vi "kloehn_error.vi"(3 "kloehn session in":T1={"VISA resource out"="COM12", "error out"={"status"=FALSE, "code"=0, "source"=""}}) -> (0 "error?":bool, 1 "kloehn session out":T1={"VISA resource out"="COM12", "error out"={"status"=FALSE, "code"=0, "source"=""}})   [LabVIEW 2010]
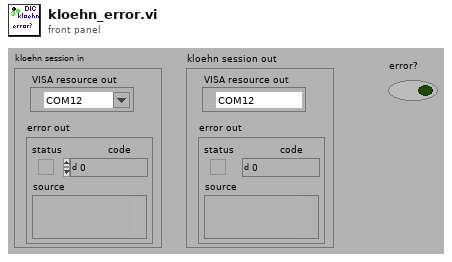
[diagram p1: front panel]
types:
  T1 = cluster{"VISA resource out":refnum<visa-resource-name>, "error out":errorcluster}
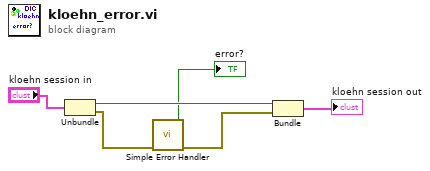
[diagram p0: block diagram]
diagram:
  n1 = Unbundle("kloehn session in") -> ("VISA resource out"=w4:refnum<visa-resource-name>, "error out"=w3:errorcluster)
  n2 = call <vilib>:"Simple Error Handler.vi"("error in (no error)"=w3) -> ("error?"=→"error?":bool, "error out"=w2:errorcluster)  [unwired: 4 in, 3 out]
  n3 = Bundle("VISA resource out"=w4, "error out"=w2) -> (→"kloehn session out":T1)  [unwired: 1 in]
